vi "Draw SliveAvg line.vi"(8 "error in (no error)":errorcluster, 9 "Coords-end":T2, 10 "Coords-start":T2, 11 "PlotAreaBounds":T1) -> (0 "error out":errorcluster, 3 "picture":picture)   [LabVIEW 2021, in "RocketPlot.lvlib"]
uses:
  RocketPlot.lvlib
  <vilib>/Utility/miscctls.llb/LVPoint32TypeDef.ctl
  <vilib>/Utility/miscctls.llb/LVRectTypeDef.ctl
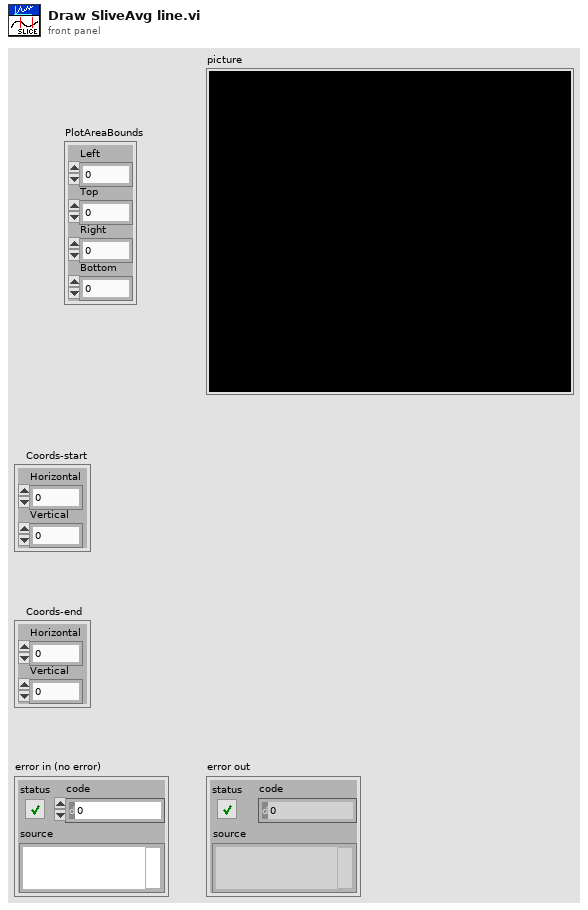
[diagram p1: front panel]
types:
  T1 = typedef "LVRectTypeDef.ctl" = cluster{"Left":i16, "Top":i16, "Right":i16, "Bottom":i16}
  T2 = typedef "LVPoint32TypeDef.ctl" = cluster{"Horizontal":i32, "Vertical":i32}
  T3 = cluster{"left":i16, "top":i16, "right":i16, "bottom":i16}
  T4 = cluster{"Width":u16, "Style":enum32{"Solid", "Dash", "Dot", "DashDot", "DashDotDot"}}
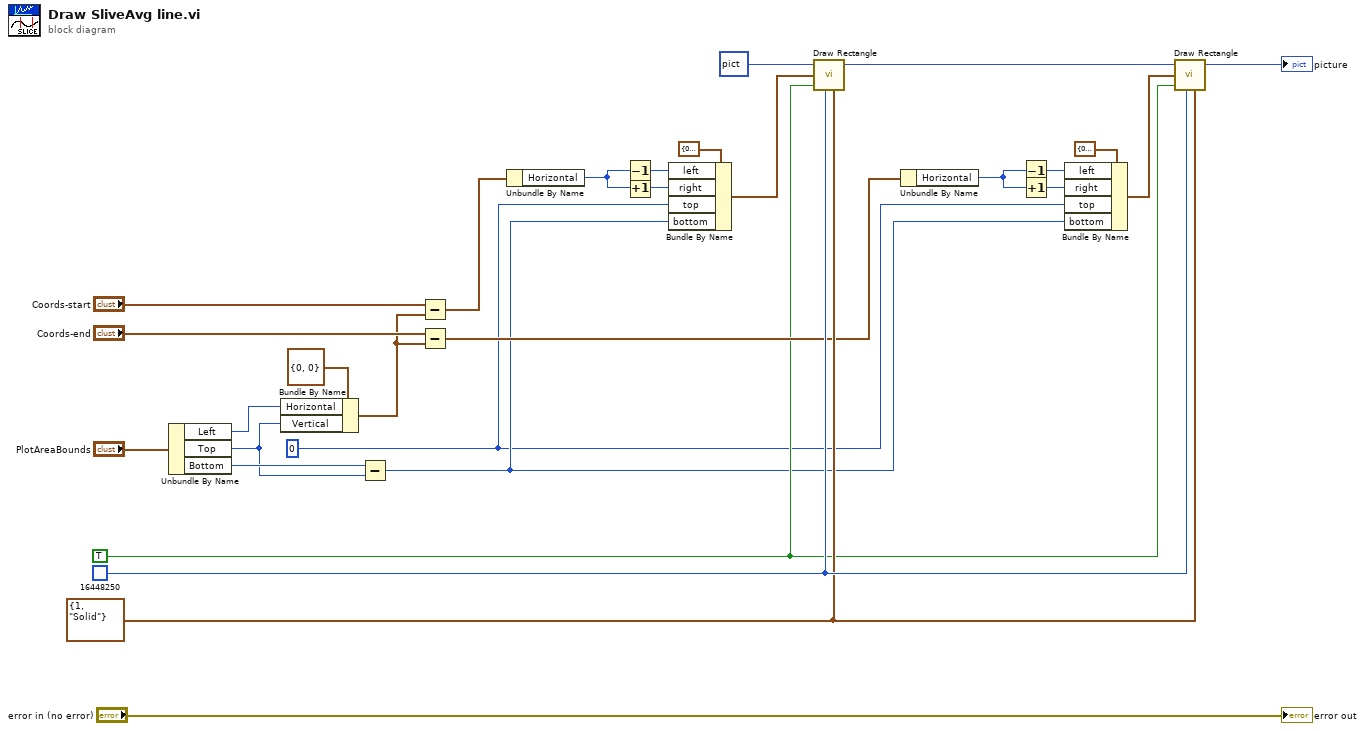
[diagram p0: block diagram]
diagram:
  w1 = i16 0 ("x-y")
  w5 = TRUE ("fill?(F)")
  w13 = u32 16448250 ("color(black)")
  w12 = T4 {"Width"=1, "Style"=enum."Solid"} ("pen")
  n1 = Unbundle By Name("PlotAreaBounds") -> ("Left"=w20:i16, "Top"=w3:i16, "Bottom"=w4:i16)
  n2 = Bundle By Name(cluster=T2 {"Horizontal"=0, "Vertical"=0} ("Coords"), "Horizontal"=w20, "Vertical"=w3) -> (w18:T2)
  n3 = Subtract(x=w4, y=w3) -> (x-y=w2:i16)
  n4 = Subtract(x="Coords-start", y=w18) -> (x-y=w24:T2)
  n5 = Subtract(x="Coords-end", y=w18) -> (x-y=w7:T2)
  n6 = Unbundle By Name(w24) -> ("Horizontal"=w23:i32)
  n7 = Decrement(x=w23) -> (x-1=w22:i32)
  n8 = Increment(x=w23) -> (x+1=w16:i32)
  n9 = Bundle By Name(cluster=T3 {"left"=0, "top"=0, "right"=0, "bottom"=0} ("rect"), "left"=w22, "right"=w16, "top"=w1, "bottom"=w2) -> (w17:T3)
  n10 = call <vilib>:"Draw Rectangle.vi"("picture"=picture data[5B], "rect"=w17, "fill?(F)"=w5, "color(black)"=w13, "pen"=w12) -> ("new picture"=w15:picture)  [unwired: 4 in]
  n11 = Unbundle By Name(w7) -> ("Horizontal"=w9:i32)
  n12 = Decrement(x=w9) -> (x-1=w10:i32)
  n13 = Increment(x=w9) -> (x+1=w11:i32)
  n14 = Bundle By Name(cluster=T3 {"left"=0, "top"=0, "right"=0, "bottom"=0} ("rect"), "left"=w10, "right"=w11, "top"=w1, "bottom"=w2) -> (w6:T3)
  n15 = call <vilib>:"Draw Rectangle.vi"("picture"=w15, "rect"=w6, "fill?(F)"=w5, "color(black)"=w13, "pen"=w12) -> ("new picture"=→"picture":picture)  [unwired: 4 in]
  "error out" <- "error in (no error)"
